vi "Special Test UI.vi"() -> ()   [LabVIEW 2025, in "Special Test.lvlib" / "Special Test.lvclass"]
doc: "Copyright 2017 National Instruments Corporation\n\nLicensed under the Apache License, Version 2.0 (the \"License\"); you may not use this file except in compliance with the License. You may obtain a copy of the License at http://www.apache.org/licenses/LICENSE-2.0\nUnless required by applicable law or agreed to in writing, software distributed under the License is distributed on an \"AS IS\" BASIS, WITHOUT WARRANTIES OR CONDITIONS OF ANY KIND, either express or implied. See the License for the specific language governing permissions and limitations under the License."
uses:
  Special Test.lvclass
  Special Test configuration/Test Info.ctl
  Users/Public/Documents/Sandia National Labs/TSS Plugin/CEF.lvlibp/Node/UserEventRef.ctl
  Users/Public/Documents/Sandia National Labs/TSS Plugin/CEF.lvlibp/Node/mainQref.ctl
  Users/Public/Documents/Sandia National Labs/TSS Plugin/CEF.lvlibp/Node/NodeRef.ctl
  Users/Public/Documents/Sandia National Labs/TSS Plugin/CEF.lvlibp/Node/CEF_Node.lvclass
  C:/Users/Public/Documents/Sandia National Labs/TSS Plugin/CEF.lvlibp/Node/CEF_Node.lvclass
  Special Test.lvclass/Special Test.ctl
  Special Test configuration/Special Test configuration.lvclass/Special Test configuration.ctl
  Special Test configuration/Read Test Info.vi
  Special Test configuration/Write Test Info.vi
  <vilib>/Utility/error.llb/Trim Whitespace One-Sided.vi
  Special Test configuration/Special Test configuration.lvclass
panel:
  in  "node ref":T1
  in  "Test Info":T2={"General"={"Location"="840/176", "Operator"="JLee"}, "Doc"={"Shorthand Test Name"="RVIT1", "MRS Code"="EI020", "P6 Test Activity Name"="JST87NE_RVIT1", "Test Plan"="Added the Version section.", "Wiring Diagram"="HW Configuration"}, "Test Setup"={"Series"="N/A", "Test Code"="N/A", "Test Group"="SNL/NM", "Config Type"="Jung.L"}, "Run"={"Temperature"="Ambient", "Voltage"="Norminal", "Attempt"=1, "Test Run"="3AxxxxxA", "Pre-Test Notes"="TK3AxxxxA", "Source Code"="900", "During Environment"="1", "Enable Dropouts"=FALSE}} {"Run"."Attempt" min=1}
  in  "main queue":T3
  in  "user event":T4
  # "(Select the Shorthand Test Name )"
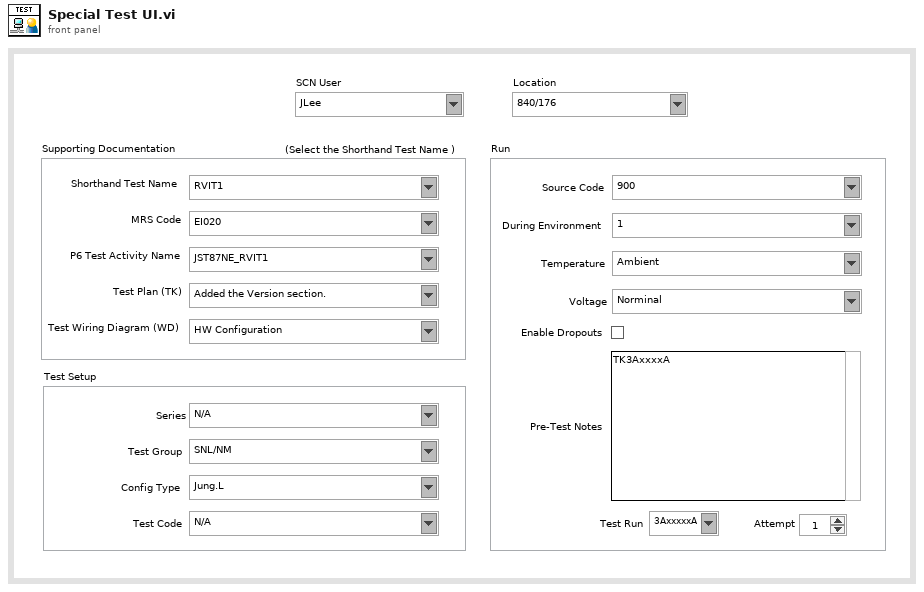
[diagram p1: front panel]
types:
  T1 = typedef "CEF.lvlibp/CEF_Node.lvclass/NodeRef.ctl" = refnum<data-value>
  T2 = typedef "Special Test.lvlib/Special Test configuration.lvclass/Test Info.ctl" = cluster{"General":cluster{"Location":string, "Operator":string}, "Doc":cluster{"Shorthand Test Name":string, "MRS Code":string, "P6 Test Activity Name":string, "Test Plan":string, "Wiring Diagram":string}, "Test Setup":cluster{"Series":string, "Test Code":string, "Test Group":string, "Config Type":string}, "Run":cluster{"Temperature":string, "Voltage":string, "Attempt":u32, "Test Run":string, "Pre-Test Notes":string, "Source Code":string, "During Environment":string, "Enable Dropouts":bool}}
  T3 = typedef "CEF.lvlibp/CEF_Node.lvclass/mainQref.ctl" = refnum<queue>
  T4 = typedef "CEF.lvlibp/CEF_Node.lvclass/UserEventRef.ctl" = refnum<user-event>
  T5 = cluster{"[0]":string, "[1]":string, "[2]":string, "[3]":string, "[4]":string}
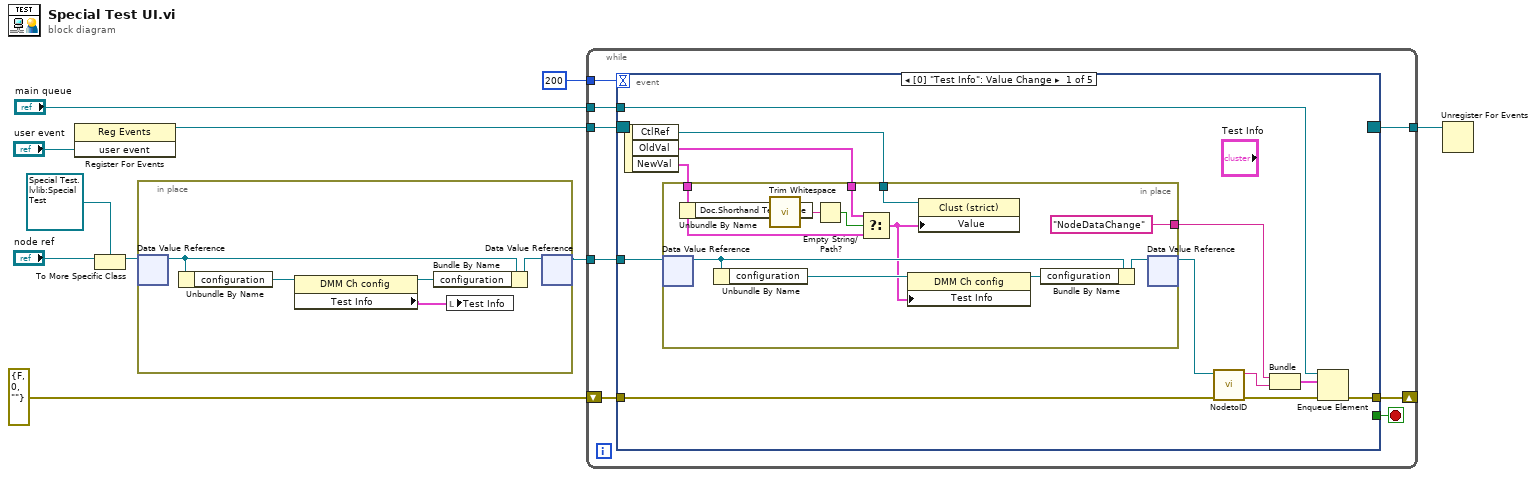
[diagram p0: block diagram]
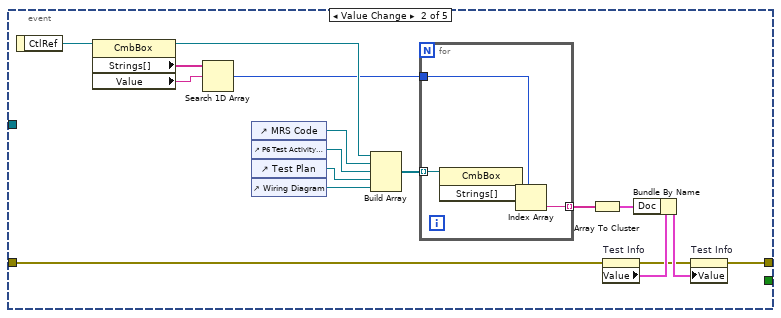
[diagram p2: hidden frame]
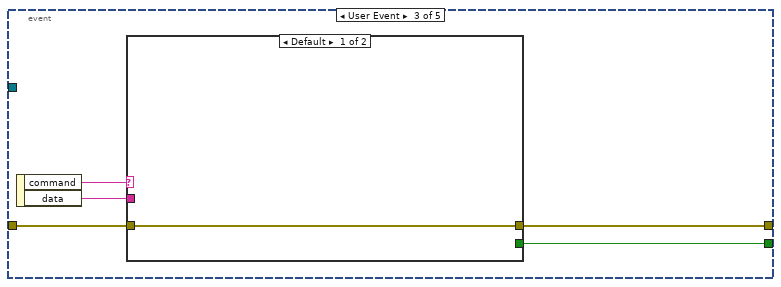
[diagram p3: hidden frame]
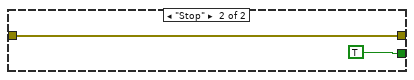
[diagram p4: hidden frame]
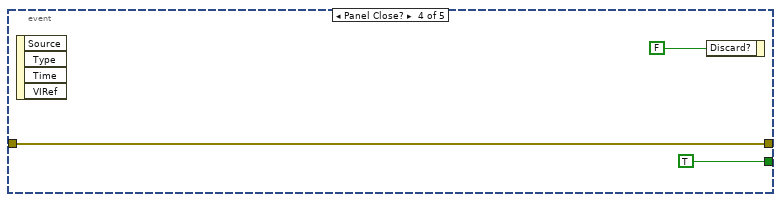
[diagram p5: hidden frame]
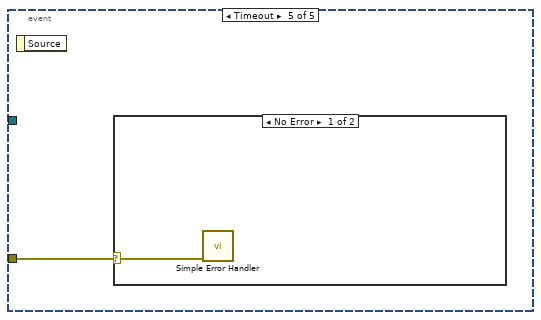
[diagram p6: hidden frame]
diagram:
  n1 = register-events("user event") -> (reference out=w9:refnum<event-registration>)  [unwired: 2 in, 1 out]
  n2 = To More Specific Class(target class=refnum<data-value> refnum ("data value reference"), reference="node ref") -> (specific class reference=w5:refnum<data-value>)  [unwired: 1 in, 1 out]
  n3 = in-place {
    # "Initialize the front panel controls when loaded"
    n4 = in-place-dvr #1(w5) -> (w15:refnum<class "Special Test.lvclass">)  [unwired: 1 out]
    n5 = Unbundle By Name(w15) -> ("configuration"=w14:refnum<class "Special Test configuration.lvclass">)
    n6 = property class="DMM Ch config"(reference=w14) -> (reference out=w12:refnum<class "Special Test configuration.lvclass">, "Test Info"=w11:T2)  [unwired: 1 in, 1 out]
    n7 = Bundle By Name(cluster=w15, "configuration"=w12) -> (w13:refnum<class "Special Test.lvclass">)
    n8 = local write "Test Info"(w11) -> ()
    n9 = in-place-dvr #1(w13) -> (w4:refnum<data-value>)  [unwired: 1 out]
  }
  n10 = while {
    tunnel: w9 -> [w23]
    tunnel: [w22] -> w8
    shift-right: [w20] -> _
    shift-left: errorcluster {"status"=FALSE, "code"=0, "source"=""} ("error in (no error)") -> [w19]
    tunnel: "main queue" -> [w18]
    tunnel: w4 -> [w17]
    tunnel: 200 -> [w16]
    stop <- w21 stop-if-true
    n11 = event shown="[0] \"Test Info\": Value Change" {
      selector: w23 -> [_ _ _ _ _]
      dyn-events: [_ _ _ _ _] -> w22
      timeout: w16 -> [_ _ _ _ _]
      tunnel: [_ _ w73 TRUE _] -> w21
      tunnel: [w27 w48 w71 w78 _] -> w20
      tunnel: w19 -> [w28 w50 w72 w78 w80]
      tunnel: w18 -> [w26 _ _ _ _]
      tunnel: w17 -> [w32 _ _ _ _]
      event Value Change {
        n12 = event-data() -> ("CtlRef"=w33:refnum<vi>, "OldVal"=w34:T2, "NewVal"=w35:T2)  [unwired: 1 in]
        n13 = in-place {
          in-place-border: w34 -> [w44]
          in-place-border: w33 -> [w43]
          in-place-border: w35 -> [w39]
          in-place-border: ["NodeDataChange" ("Message Name")] -> w25
          n14 = in-place-dvr #2(w32) -> (w47:refnum<class "Special Test.lvclass">)  [unwired: 1 out]
          n15 = Unbundle By Name(w39) -> ("Doc.Shorthand Test Name"=w38:string)
          n16 = Unbundle By Name(w47) -> ("configuration"=w42:refnum<class "Special Test configuration.lvclass">)
          n17 = call <vilib>:"Trim Whitespace.vi"("string"=w38) -> ("trimmed string"=w41:string)  [unwired: 1 in]
          n18 = Empty String/Path?(string/path=w41) -> (empty?=w40:bool)
          n19 = Select(t=w44, s=w40, f=w39) -> (s? t:f=w36:T2)
          n20 = property class="DMM Ch config"(reference=w42, "Test Info"=w36) -> (reference out=w46:refnum<class "Special Test configuration.lvclass">)  [unwired: 1 in, 1 out]
          n21 = property class="Clust (strict)"(reference=w43, "Value"=w36) -> ()  [unwired: 1 in, 2 out]
          n22 = Bundle By Name(cluster=w47, "configuration"=w46) -> (w45:refnum<class "Special Test.lvclass">)
          n23 = in-place-dvr #2(w45) -> (w24:refnum<data-value>)  [unwired: 1 out]
        }
        n24 = call "NodetoID.vi"("error in"=w28, "node ref"=w24) -> ("error out"=w31:errorcluster, "ID"=w29:string)  [unwired: 8 in]
        n25 = Bundle("Message Name"=w25, "ID"=w29) -> (w30:cluster{"Message Name":string, "ID":string})  [unwired: 1 in]
        n26 = Enqueue Element(queue=w26, element=w30, error in (no error)=w31) -> (error out=w27:errorcluster)  [unwired: 1 in, 2 out]
      }
      event Value Change {
        n27 = event-data() -> ("CtlRef"=w58:refnum<vi>)  [unwired: 1 in]
        n28 = property class="CmbBox"(reference=w58) -> (reference out=w57:refnum<vi>, "Strings[]"=w64:string[], "Value"=w63:string)  [unwired: 1 in, 1 out]
        n29 = Search 1D Array(1D array=w64, element=w63) -> (index of element=w55:i32)  [unwired: 1 in]
        n30 = control-ref of="MRS Code"() -> (w62:refnum<vi>)
        n31 = control-ref of="P6 Test Activity Name"() -> (w61:refnum<vi>)
        n32 = control-ref of="Test Plan"() -> (w60:refnum<vi>)
        n33 = control-ref of="Wiring Diagram"() -> (w59:refnum<vi>)
        n34 = Build Array(w57, w62, w61, w60, w59) -> (w56:refnum<vi>[])
        n35 = for {
          tunnel: w56 -> [w67] mode=indexing
          tunnel: w55 -> [w66]
          tunnel: [w65] -> w54 mode=indexing
          n36 = property class="CmbBox"(reference=w67) -> ("Strings[]"=w68:string[])  [unwired: 1 in, 2 out]
          n37 = Index Array(array=w68, index=w66) -> (element=w65:string)
        }
        n38 = Array To Cluster(array=w54) -> (cluster=w53:T5)
        n39 = property on="Test Info" class="Clust (strict)"(error in=w50) -> (error out=w49:errorcluster, "Value"=w52:T2)  [unwired: 1 in, 1 out]
        n40 = Bundle By Name(cluster=w52, "Doc"=w53) -> (w51:T2)
        n41 = property on="Test Info" class="Clust (strict)"(error in=w49, "Value"=w51) -> (error out=w48:errorcluster)  [unwired: 1 in, 1 out]
      }
      event User Event {
        n42 = event-data() -> ("command"=w69:string, "data"=w70:string)  [unwired: 1 in]
        n43 = case shown="Default" w69 {
          tunnel: w70 -> [_ _]
          tunnel: [_ TRUE] -> w73
          tunnel: w72 -> [w74 w75]
          tunnel: [w74 w75] -> w71
          frame Default {
          }
          frame "Stop" {
          }
        }
      }
      event Panel Close? {
        n44 = event-data() -> ()  [unwired: 1 in, 4 out]
        n45 = event-data("Discard?"=FALSE) -> ()  [unwired: 1 in, 1 out]
      }
      event Timeout {
        n46 = event-data() -> ()  [unwired: 1 in, 1 out]
        n47 = case shown="No Error" w80 {
          selector: w80 -> [w81 _]
          frame No Error {
            n48 = call <vilib>:"Simple Error Handler.vi"("error in (no error)"=w81) -> ()  [unwired: 4 in, 5 out]
          }
          frame Error {
          }
        }
      }
    }
  }
  n49 = Unregister For Events(event registration refnum=w8) -> ()  [unwired: 1 in, 1 out]
